vi "SLSC Convert Items - Variant to String.vi"(0 "dataType":string, 1 "format string":string="%#_12g", 5 "value":variant, 7 "min":variant, 9 "max":variant, 12 "string enums":T2(array[cluster])) -> (4 "Output data type":string, 6 "string offline data value":string, 8 "string min":string, 10 "string max":string, 14 "data_range":string)   [LabVIEW 2017, in "SLSC Tree Control.lvlib"]
doc: "Converts all of the item elements from variant into strings."
uses:
  SLSC Tree Control.lvlib
  Ctrl/EnumValue.ctl
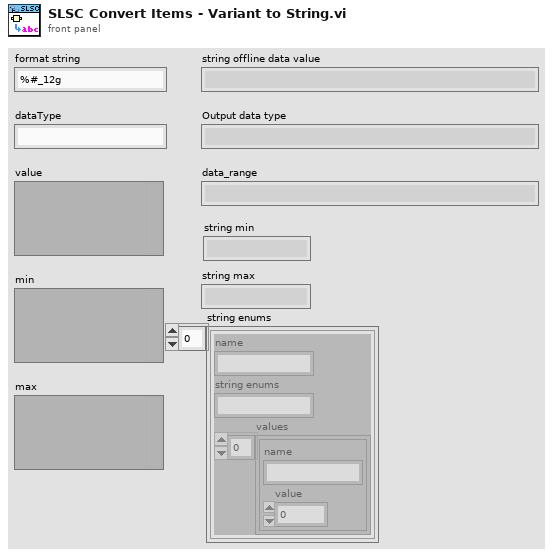
[diagram p1: front panel]
types:
  T1 = typedef "EnumValue.ctl" = cluster{"name":string, "value":i32}
  T2 = cluster{"name":string, "string enums":string, "values":T1[]}[]
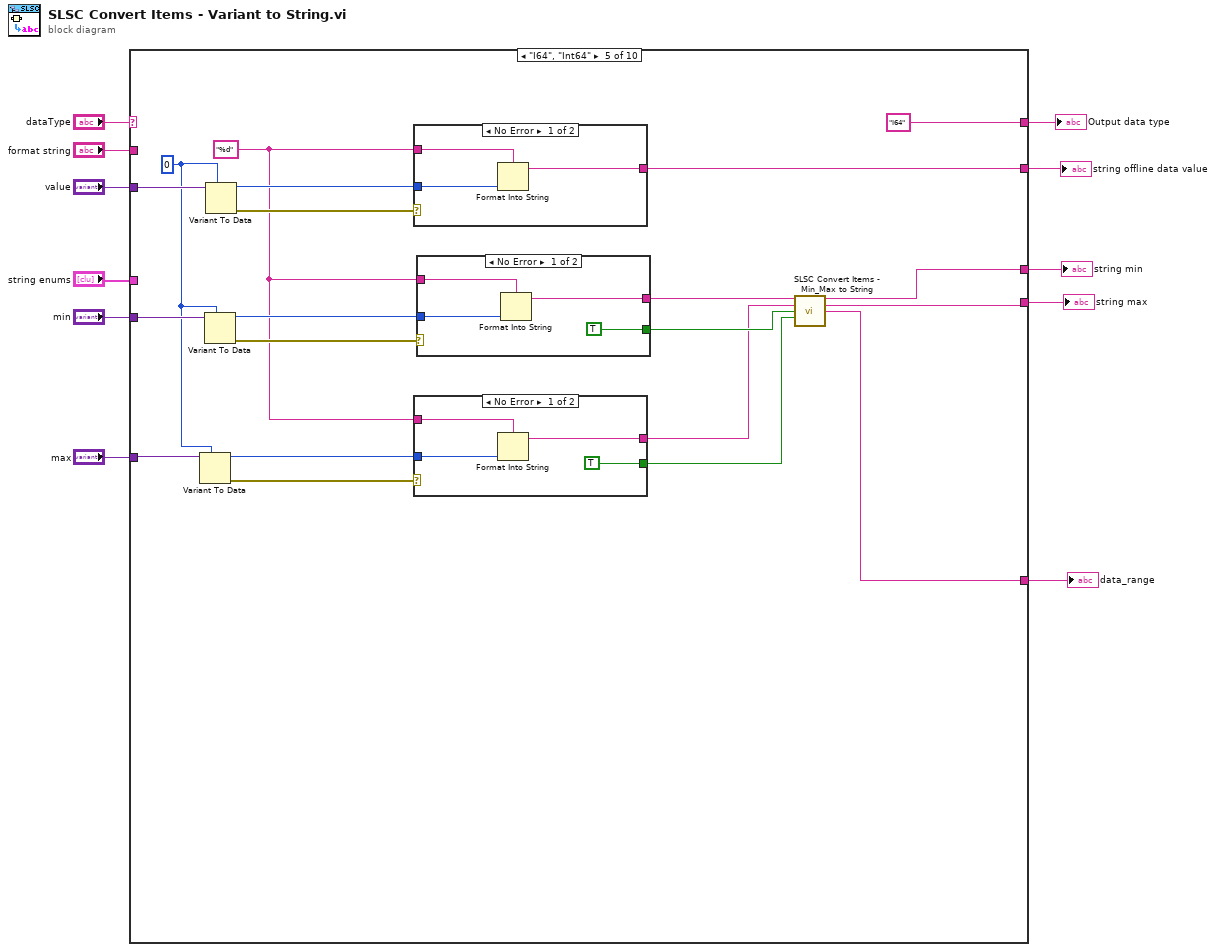
[diagram p0: block diagram]
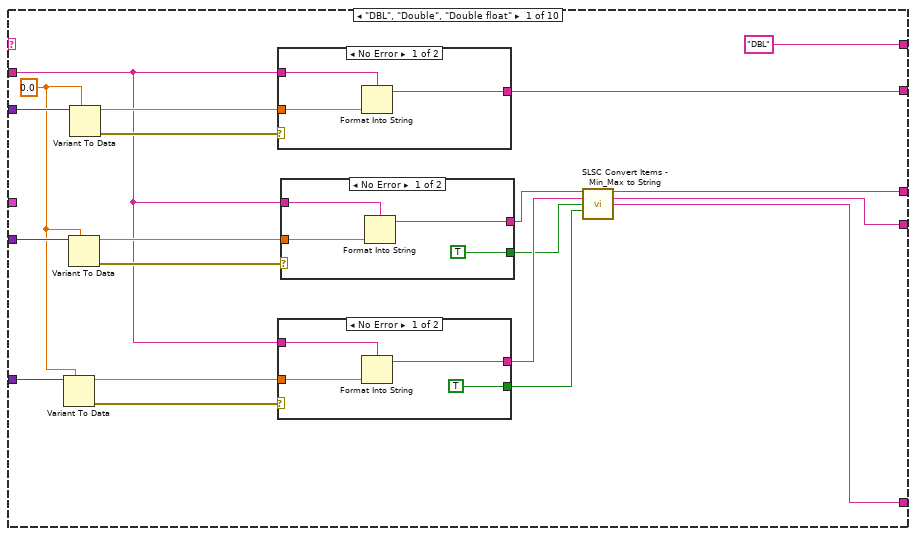
[diagram p2: hidden frame]
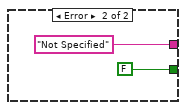
[diagram p3: hidden frame]
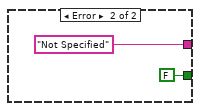
[diagram p4: hidden frame]
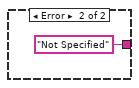
[diagram p5: hidden frame]
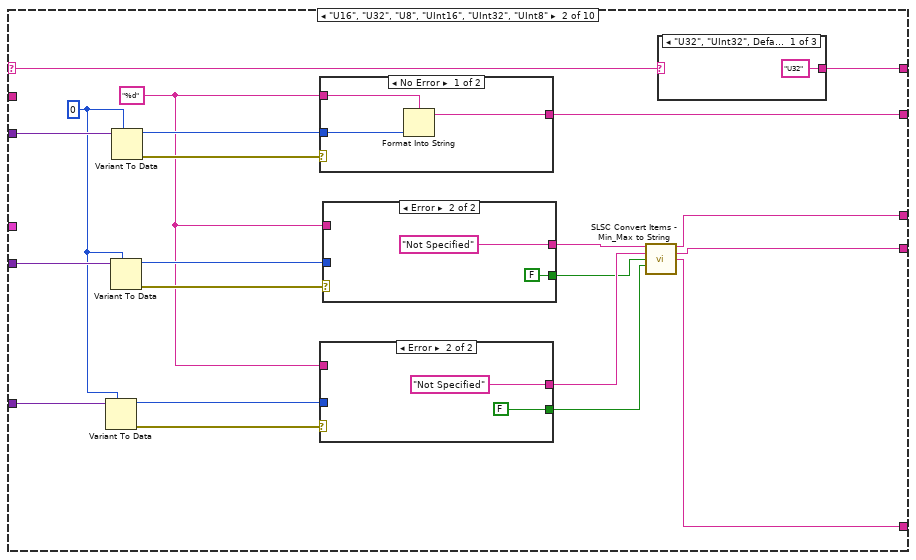
[diagram p6: hidden frame]
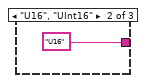
[diagram p7: hidden frame]
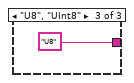
[diagram p8: hidden frame]
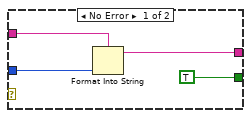
[diagram p9: hidden frame]
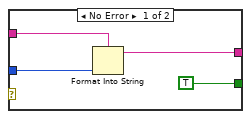
[diagram p10: hidden frame]
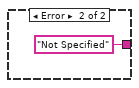
[diagram p11: hidden frame]
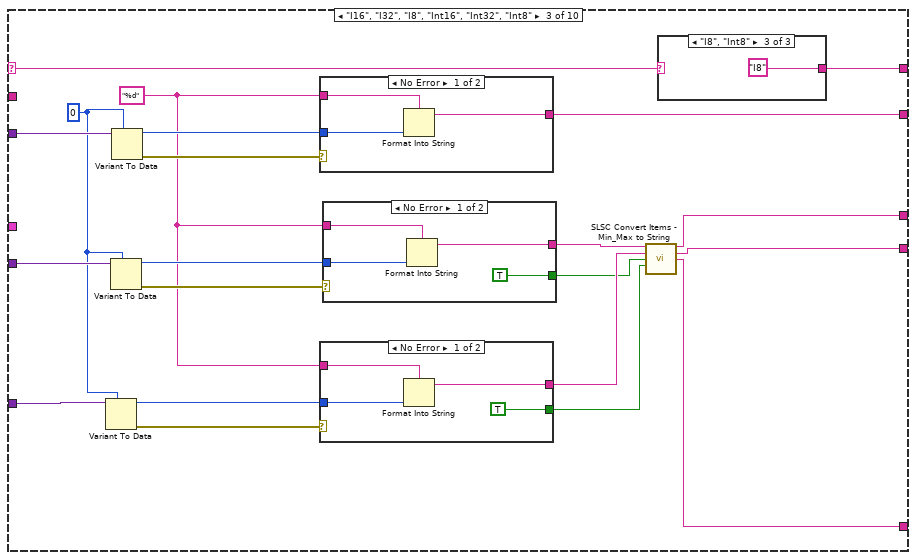
[diagram p12: hidden frame]
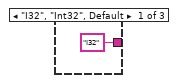
[diagram p13: hidden frame]
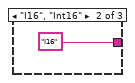
[diagram p14: hidden frame]
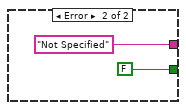
[diagram p15: hidden frame]
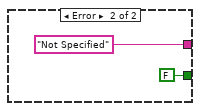
[diagram p16: hidden frame]
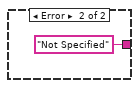
[diagram p17: hidden frame]
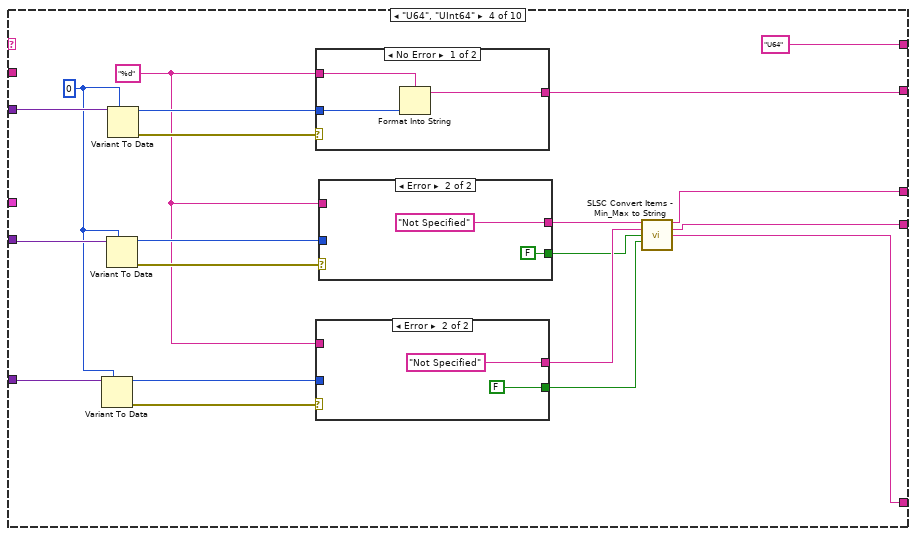
[diagram p18: hidden frame]
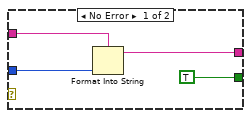
[diagram p19: hidden frame]
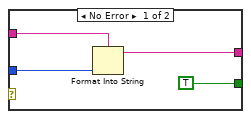
[diagram p20: hidden frame]
diagram:
  n1 = case shown="\"I64\", \"Int64\"" "dataType" {
    selector: "dataType" -> [_ w51 w91 _ _ _ w242 w248 w321 w403]
    tunnel: "value" -> [w31 w58 w98 w141 w174 w216 w241 w249 w322 w406]
    tunnel: [w23 w55 w95 w138 w167 w217 w240 w244 w317 w404] -> w4
    tunnel: ["DBL" w50 w90 "U64" "I64" "Bool" w242 w248 w321 w403] -> w9
    tunnel: "min" -> [w29 w57 w97 w140 w173 w212 _ w246 w319 w401]
    tunnel: "max" -> [w28 w56 w96 w139 w172 w210 _ w245 w318 w399]
    tunnel: [w26 w54 w94 w133 w182 w205 _ _ _ _] -> w6
    tunnel: [w25 w53 w93 w132 w181 w204 _ _ _ _] -> w5
    tunnel: "format string" -> [w12 _ _ _ _ _ _ _ _ _]
    tunnel: "string enums" -> [_ _ _ _ _ _ _ w247 w320 w405]
    tunnel: [w27 w52 w92 w131 w183 w203 _ w243 w316 w396] -> w11
    frame "DBL", "Double", "Double float" {
      w13 = 0.0
      n2 = Variant To Data(type=w13, Variant=w28) -> (data=w18:dbl, error out=w19:errorcluster)  [unwired: 1 in]
      n3 = Variant To Data(type=w13, Variant=w29) -> (data=w20:dbl, error out=w21:errorcluster)  [unwired: 1 in]
      n4 = Variant To Data(type=w13, Variant=w31) -> (data=w30:dbl, error out=w22:errorcluster)  [unwired: 1 in]
      n5 = case shown="No Error" w22 {
        tunnel: w30 -> [w46 _]
        tunnel: w12 -> [w45 _]
        tunnel: [w44 "Not Specified"] -> w23
        frame No Error {
          n6 = Format Into String(format string=w45, w46) -> (resulting string=w44:string)  [unwired: 2 in, 1 out]
        }
        frame Error {
        }
      }
      n7 = case shown="No Error" w19 {
        tunnel: w18 -> [w35 _]
        tunnel: w12 -> [w34 _]
        tunnel: [w33 "Not Specified"] -> w16
        tunnel: [TRUE ("min?") FALSE ("min?")] -> w14
        frame No Error {
          n8 = Format Into String(format string=w34, w35) -> (resulting string=w33:string)  [unwired: 2 in, 1 out]
        }
        frame Error {
        }
      }
      n9 = case shown="No Error" w21 {
        tunnel: w20 -> [w41 _]
        tunnel: w12 -> [w40 _]
        tunnel: [w39 "Not Specified"] -> w17
        tunnel: [TRUE ("min?") FALSE ("min?")] -> w15
        frame No Error {
          n10 = Format Into String(format string=w40, w41) -> (resulting string=w39:string)  [unwired: 2 in, 1 out]
        }
        frame Error {
        }
      }
      n11 = call "SLSC Convert Items - Min_Max to String.vi"("minimum"=w17, "maximum"=w16, "min?"=w15, "max?"=w14) -> ("minimum out"=w26:string, "maximum out"=w25:string, "minmax string"=w27:string)  [unwired: 9 in]
    }
    frame "U16", "U32", "U8", "UInt16", "UInt32", "UInt8" {
      w48 = "%d" ("format string")
      w49 = u32 0
      n12 = Variant To Data(type=w49, Variant=w56) -> (data=w63:u32, error out=w64:errorcluster)  [unwired: 1 in]
      n13 = Variant To Data(type=w49, Variant=w57) -> (data=w65:u32, error out=w66:errorcluster)  [unwired: 1 in]
      n14 = Variant To Data(type=w49, Variant=w58) -> (data=w68:u32, error out=w67:errorcluster)  [unwired: 1 in]
      n15 = case shown="No Error" w67 {
        tunnel: w68 -> [w86 _]
        tunnel: w48 -> [w85 _]
        tunnel: [w84 "Not Specified"] -> w55
        frame No Error {
          n16 = Format Into String(format string=w85, w86) -> (resulting string=w84:string)  [unwired: 2 in, 1 out]
        }
        frame Error {
        }
      }
      n17 = case shown="Error" w64 {
        tunnel: w63 -> [w75 _]
        tunnel: w48 -> [w74 _]
        tunnel: [w73 "Not Specified"] -> w61
        tunnel: [TRUE ("min?") FALSE ("min?")] -> w59
        frame No Error {
          n18 = Format Into String(format string=w74, w75) -> (resulting string=w73:string)  [unwired: 2 in, 1 out]
        }
        frame Error {
        }
      }
      n19 = case shown="Error" w66 {
        tunnel: w65 -> [w81 _]
        tunnel: w48 -> [w80 _]
        tunnel: [w79 "Not Specified"] -> w62
        tunnel: [TRUE ("min?") FALSE ("min?")] -> w60
        frame No Error {
          n20 = Format Into String(format string=w80, w81) -> (resulting string=w79:string)  [unwired: 2 in, 1 out]
        }
        frame Error {
        }
      }
      n21 = call "SLSC Convert Items - Min_Max to String.vi"("minimum"=w62, "maximum"=w61, "min?"=w60, "max?"=w59) -> ("minimum out"=w54:string, "maximum out"=w53:string, "minmax string"=w52:string)  [unwired: 9 in]
      n22 = case shown="\"U32\", \"UInt32\", Default" w51 {
        tunnel: ["U32" "U16" "U8"] -> w50
        frame "U32", "UInt32", Default {
        }
        frame "U16", "UInt16" {
        }
        frame "U8", "UInt8" {
        }
      }
    }
    frame "I16", "I32", "I8", "Int16", "Int32", "Int8" {
      w88 = "%d" ("format string")
      w89 = 0
      n23 = Variant To Data(type=w89, Variant=w96) -> (data=w103:i32, error out=w104:errorcluster)  [unwired: 1 in]
      n24 = Variant To Data(type=w89, Variant=w97) -> (data=w105:i32, error out=w106:errorcluster)  [unwired: 1 in]
      n25 = Variant To Data(type=w89, Variant=w98) -> (data=w108:i32, error out=w107:errorcluster)  [unwired: 1 in]
      n26 = case shown="No Error" w107 {
        tunnel: w108 -> [w126 _]
        tunnel: w88 -> [w125 _]
        tunnel: [w124 "Not Specified"] -> w95
        frame No Error {
          n27 = Format Into String(format string=w125, w126) -> (resulting string=w124:string)  [unwired: 2 in, 1 out]
        }
        frame Error {
        }
      }
      n28 = case shown="No Error" w104 {
        tunnel: w103 -> [w115 _]
        tunnel: w88 -> [w114 _]
        tunnel: [w113 "Not Specified"] -> w101
        tunnel: [TRUE ("min?") FALSE ("min?")] -> w99
        frame No Error {
          n29 = Format Into String(format string=w114, w115) -> (resulting string=w113:string)  [unwired: 2 in, 1 out]
        }
        frame Error {
        }
      }
      n30 = case shown="No Error" w106 {
        tunnel: w105 -> [w121 _]
        tunnel: w88 -> [w120 _]
        tunnel: [w119 "Not Specified"] -> w102
        tunnel: [TRUE ("min?") FALSE ("min?")] -> w100
        frame No Error {
          n31 = Format Into String(format string=w120, w121) -> (resulting string=w119:string)  [unwired: 2 in, 1 out]
        }
        frame Error {
        }
      }
      n32 = call "SLSC Convert Items - Min_Max to String.vi"("minimum"=w102, "maximum"=w101, "min?"=w100, "max?"=w99) -> ("minimum out"=w94:string, "maximum out"=w93:string, "minmax string"=w92:string)  [unwired: 9 in]
      n33 = case shown="\"I8\", \"Int8\"" w91 {
        tunnel: ["I32" "I16" "I8"] -> w90
        frame "I32", "Int32", Default {
        }
        frame "I16", "Int16" {
        }
        frame "I8", "Int8" {
        }
      }
    }
    frame "U64", "UInt64" {
      w128 = "%d" ("format string")
      w129 = u64 0
      n34 = Variant To Data(type=w129, Variant=w139) -> (data=w142:u64, error out=w143:errorcluster)  [unwired: 1 in]
      n35 = Variant To Data(type=w129, Variant=w140) -> (data=w144:u64, error out=w145:errorcluster)  [unwired: 1 in]
      n36 = Variant To Data(type=w129, Variant=w141) -> (data=w147:u64, error out=w146:errorcluster)  [unwired: 1 in]
      n37 = case shown="No Error" w146 {
        tunnel: w147 -> [w162 _]
        tunnel: w128 -> [w161 _]
        tunnel: [w160 "Not Specified"] -> w138
        frame No Error {
          n38 = Format Into String(format string=w161, w162) -> (resulting string=w160:string)  [unwired: 2 in, 1 out]
        }
        frame Error {
        }
      }
      n39 = case shown="Error" w143 {
        tunnel: w142 -> [w151 _]
        tunnel: w128 -> [w150 _]
        tunnel: [w149 "Not Specified"] -> w136
        tunnel: [TRUE ("min?") FALSE ("min?")] -> w134
        frame No Error {
          n40 = Format Into String(format string=w150, w151) -> (resulting string=w149:string)  [unwired: 2 in, 1 out]
        }
        frame Error {
        }
      }
      n41 = case shown="Error" w145 {
        tunnel: w144 -> [w157 _]
        tunnel: w128 -> [w156 _]
        tunnel: [w155 "Not Specified"] -> w137
        tunnel: [TRUE ("min?") FALSE ("min?")] -> w135
        frame No Error {
          n42 = Format Into String(format string=w156, w157) -> (resulting string=w155:string)  [unwired: 2 in, 1 out]
        }
        frame Error {
        }
      }
      n43 = call "SLSC Convert Items - Min_Max to String.vi"("minimum"=w137, "maximum"=w136, "min?"=w135, "max?"=w134) -> ("minimum out"=w133:string, "maximum out"=w132:string, "minmax string"=w131:string)  [unwired: 9 in]
    }
    frame "I64", "Int64" {
      w164 = "%d" ("format string")
      w165 = i64 0
      n44 = Variant To Data(type=w165, Variant=w172) -> (data=w175:i64, error out=w176:errorcluster)  [unwired: 1 in]
      n45 = Variant To Data(type=w165, Variant=w173) -> (data=w177:i64, error out=w178:errorcluster)  [unwired: 1 in]
      n46 = Variant To Data(type=w165, Variant=w174) -> (data=w180:i64, error out=w179:errorcluster)  [unwired: 1 in]
      n47 = case shown="No Error" w179 {
        tunnel: w180 -> [w198 _]
        tunnel: w164 -> [w197 _]
        tunnel: [w196 "Not Specified"] -> w167
        frame No Error {
          n48 = Format Into String(format string=w197, w198) -> (resulting string=w196:string)  [unwired: 2 in, 1 out]
        }
        frame Error {
        }
      }
      n49 = case shown="No Error" w176 {
        tunnel: w175 -> [w187 _]
        tunnel: w164 -> [w186 _]
        tunnel: [w185 "Not Specified"] -> w169
        tunnel: [TRUE ("min?") FALSE ("min?")] -> w168
        frame No Error {
          n50 = Format Into String(format string=w186, w187) -> (resulting string=w185:string)  [unwired: 2 in, 1 out]
        }
        frame Error {
        }
      }
      n51 = case shown="No Error" w178 {
        tunnel: w177 -> [w193 _]
        tunnel: w164 -> [w192 _]
        tunnel: [w191 "Not Specified"] -> w171
        tunnel: [TRUE ("min?") FALSE ("min?")] -> w170
        frame No Error {
          n52 = Format Into String(format string=w192, w193) -> (resulting string=w191:string)  [unwired: 2 in, 1 out]
        }
        frame Error {
        }
      }
      n53 = call "SLSC Convert Items - Min_Max to String.vi"("minimum"=w171, "maximum"=w169, "min?"=w170, "max?"=w168) -> ("minimum out"=w182:string, "maximum out"=w181:string, "minmax string"=w183:string)  [unwired: 9 in]
    }
    frame "Bool", "Boolean" {
      n54 = Equal?(x=w216, y=variant) -> (x = y?=w214:bool)
      n55 = Equal?(x=w210, y=variant) -> (x = y?=w207:bool)
      n56 = Equal?(x=w212, y=variant) -> (x = y?=w206:bool)
      n57 = Not(x=w207) -> (.not. x?=w200:bool)
      n58 = Not(x=w206) -> (.not. x?=w201:bool)
      n59 = case shown="True" w214 {
        tunnel: ["Not Specified" w236] -> w217
        tunnel: w216 -> [_ w233]
        frame True {
        }
        frame False {
          n60 = Variant To Data(type=FALSE, Variant=w233) -> (data=w234:bool)  [unwired: 1 in, 1 out]
          n61 = Select(t="True" ("data string"), s=w234, f="False" ("data string")) -> (s? t:f=w236:string)
        }
      }
      n62 = case shown="False" w207 {
        tunnel: ["Not Specified" w222] -> w208
        tunnel: w210 -> [_ w219]
        frame True {
        }
        frame False {
          n63 = Variant To Data(type=FALSE, Variant=w219) -> (data=w220:bool)  [unwired: 1 in, 1 out]
          n64 = Select(t="True" ("data string"), s=w220, f="False" ("data string")) -> (s? t:f=w222:string)
        }
      }
      n65 = case shown="False" w206 {
        tunnel: ["Not Specified" w229] -> w209
        tunnel: w212 -> [_ w226]
        frame True {
        }
        frame False {
          n66 = Variant To Data(type=FALSE, Variant=w226) -> (data=w227:bool)  [unwired: 1 in, 1 out]
          n67 = Select(t="True" ("data string"), s=w227, f="False" ("data string")) -> (s? t:f=w229:string)
        }
      }
      n68 = call "SLSC Convert Items - Min_Max to String.vi"("minimum"=w209, "maximum"=w208, "min?"=w201, "max?"=w200) -> ("minimum out"=w205:string, "maximum out"=w204:string, "minmax string"=w203:string)  [unwired: 9 in]
    }
    frame "String" {
      n69 = Variant To Data(type="" ("data string"), Variant=w241) -> (data=w240:string)  [unwired: 1 in, 1 out]
    }
    frame "NI.LEDState" {
      n70 = for {
        tunnel: w247 -> [w315] mode=indexing
        tunnel: w248 -> [w313]
        tunnel: [w310] -> w254 if=w312
        tunnel: [w312] -> _
        tunnel: [w311] -> w253
        stop <- w312 stop-if-true
        n71 = Unbundle By Name(w315) -> ("name"=w314:string, "values"=w311:T1[], "string enums"=w310:string)
        n72 = Equal?(x=w313, y=w314) -> (x = y?=w312:bool)
      }
      n73 = Variant To Data(type=0, Variant=w245) -> (data=w258:i32, error out=w260:errorcluster)  [unwired: 1 in]
      n74 = Variant To Data(type=0, Variant=w246) -> (data=w259:i32, error out=w261:errorcluster)  [unwired: 1 in]
      n75 = Unbundle By Name(w261) -> ("status"=w257:bool)
      n76 = Unbundle By Name(w260) -> ("status"=w256:bool)
      n77 = Variant To Data(type=0, Variant=w249) -> (data=w263:i32, error out=w262:errorcluster)  [unwired: 1 in]
      n78 = Or(x=w257, y=w256) -> (x .or. y?=w255:bool)
      n79 = case shown="True" w255 {
        tunnel: w257 -> [_ w277]
        tunnel: w253 -> [_ w276]
        tunnel: [w264 w274] -> w243
        tunnel: w259 -> [_ w272]
        tunnel: w256 -> [_ w267]
        tunnel: w258 -> [_ w266]
        tunnel: w254 -> [w264 _]
        frame False {
        }
        frame True {
          n80 = Not(x=w277) -> (.not. x?=w273:bool)
          n81 = Not(x=w267) -> (.not. x?=w269:bool)
          n82 = Select(t=w272, s=w273, f=-2147483648) -> (s? t:f=w270:i32)
          n83 = Select(t=w266, s=w269, f=2147483647) -> (s? t:f=w265:i32)
          n84 = for {
            tunnel: w276 -> [w285] mode=indexing
            tunnel: w270 -> [w283]
            tunnel: w265 -> [w284]
            shift-right: [w278] -> w274
            shift-left: "" -> [w279]
            n85 = Unbundle By Name(w285) -> ("name"=w280:string, "value"=w281:i32)
            n86 = In Range and Coerce(upper limit=w284, x=w281, lower limit=w283) -> (In Range?=w282:bool)  [unwired: 1 out]
            n87 = case shown="True" w282 {
              tunnel: w281 -> [_ w291]
              tunnel: w280 -> [_ w287]
              tunnel: [w286 w289] -> w278
              tunnel: w279 -> [w286 w288]
              frame False {
              }
              frame True {
                n88 = Format Into String(format string="%d", w291) -> (resulting string=w294:string)  [unwired: 2 in, 1 out]
                n89 = Concatenate Strings(w288, "[" ("string"), w294, "]" ("string"), w287, ";" ("string")) -> (w289:string)
              }
            }
          }
        }
      }
      n90 = case shown="No Error" w262 {
        tunnel: w263 -> [w297 _]
        tunnel: [w299 ""] -> w244
        tunnel: w253 -> [w298 _]
        frame No Error {
          n91 = for {
            tunnel: w298 -> [w308] mode=indexing
            tunnel: w297 -> [w306]
            tunnel: [w305] -> w296 if=w304
            stop <- w304 stop-if-true
            n92 = Unbundle By Name(w308) -> ("value"=w307:i32, "name"=w305:string)
            n93 = Equal?(x=w306, y=w307) -> (x = y?=w304:bool)
          }
          n94 = Format Into String(format string="%d", w297) -> (resulting string=w300:string)  [unwired: 2 in, 1 out]
          n95 = Concatenate Strings("[" ("string"), w300, "]" ("string"), w296) -> (w299:string)
        }
        frame Error {
        }
      }
    }
    frame "NI.EventDelay" {
      n96 = for {
        tunnel: w320 -> [w388] mode=indexing
        tunnel: w321 -> [w386]
        tunnel: [w383] -> w327 if=w385
        tunnel: [w385] -> _
        tunnel: [w384] -> w326
        stop <- w385 stop-if-true
        n97 = Unbundle By Name(w388) -> ("name"=w387:string, "values"=w384:T1[], "string enums"=w383:string)
        n98 = Equal?(x=w386, y=w387) -> (x = y?=w385:bool)
      }
      n99 = Variant To Data(type=0, Variant=w318) -> (data=w331:i32, error out=w333:errorcluster)  [unwired: 1 in]
      n100 = Variant To Data(type=0, Variant=w319) -> (data=w332:i32, error out=w334:errorcluster)  [unwired: 1 in]
      n101 = Unbundle By Name(w334) -> ("status"=w330:bool)
      n102 = Unbundle By Name(w333) -> ("status"=w329:bool)
      n103 = Variant To Data(type=0, Variant=w322) -> (data=w336:i32, error out=w335:errorcluster)  [unwired: 1 in]
      n104 = Or(x=w330, y=w329) -> (x .or. y?=w328:bool)
      n105 = case shown="True" w328 {
        tunnel: w330 -> [_ w350]
        tunnel: w326 -> [_ w349]
        tunnel: [w337 w347] -> w316
        tunnel: w332 -> [_ w345]
        tunnel: w329 -> [_ w340]
        tunnel: w331 -> [_ w339]
        tunnel: w327 -> [w337 _]
        frame False {
        }
        frame True {
          n106 = Not(x=w350) -> (.not. x?=w346:bool)
          n107 = Not(x=w340) -> (.not. x?=w342:bool)
          n108 = Select(t=w345, s=w346, f=-2147483648) -> (s? t:f=w343:i32)
          n109 = Select(t=w339, s=w342, f=2147483647) -> (s? t:f=w338:i32)
          n110 = for {
            tunnel: w349 -> [w358] mode=indexing
            tunnel: w343 -> [w356]
            tunnel: w338 -> [w357]
            shift-right: [w351] -> w347
            shift-left: "" -> [w352]
            n111 = Unbundle By Name(w358) -> ("name"=w353:string, "value"=w354:i32)
            n112 = In Range and Coerce(upper limit=w357, x=w354, lower limit=w356) -> (In Range?=w355:bool)  [unwired: 1 out]
            n113 = case shown="True" w355 {
              tunnel: w354 -> [_ w364]
              tunnel: w353 -> [_ w360]
              tunnel: [w359 w362] -> w351
              tunnel: w352 -> [w359 w361]
              frame False {
              }
              frame True {
                n114 = Format Into String(format string="%d", w364) -> (resulting string=w367:string)  [unwired: 2 in, 1 out]
                n115 = Concatenate Strings(w361, "[" ("string"), w367, "]" ("string"), w360, ";" ("string")) -> (w362:string)
              }
            }
          }
        }
      }
      n116 = case shown="No Error" w335 {
        tunnel: w336 -> [w370 _]
        tunnel: [w372 ""] -> w317
        tunnel: w326 -> [w371 _]
        frame No Error {
          n117 = for {
            tunnel: w371 -> [w381] mode=indexing
            tunnel: w370 -> [w379]
            tunnel: [w378] -> w369 if=w377
            stop <- w377 stop-if-true
            n118 = Unbundle By Name(w381) -> ("value"=w380:i32, "name"=w378:string)
            n119 = Equal?(x=w379, y=w380) -> (x = y?=w377:bool)
          }
          n120 = Format Into String(format string="%d", w370) -> (resulting string=w373:string)  [unwired: 2 in, 1 out]
          n121 = Concatenate Strings("[" ("string"), w373, "]" ("string"), w369) -> (w372:string)
        }
        frame Error {
        }
      }
    }
    frame Default {
      n122 = for {
        tunnel: w405 -> [w461] mode=indexing
        tunnel: w403 -> [w459]
        tunnel: [w456] -> w390 if=w458
        tunnel: [w458] -> _
        tunnel: [w457] -> w389
        stop <- w458 stop-if-true
        n123 = Unbundle By Name(w461) -> ("name"=w460:string, "values"=w457:T1[], "string enums"=w456:string)
        n124 = Equal?(x=w459, y=w460) -> (x = y?=w458:bool)
      }
      n125 = Variant To Data(type=0, Variant=w399) -> (data=w394:i32, error out=w397:errorcluster)  [unwired: 1 in]
      n126 = Variant To Data(type=0, Variant=w401) -> (data=w395:i32, error out=w398:errorcluster)  [unwired: 1 in]
      n127 = Unbundle By Name(w398) -> ("status"=w393:bool)
      n128 = Unbundle By Name(w397) -> ("status"=w392:bool)
      n129 = Variant To Data(type=0, Variant=w406) -> (data=w408:i32, error out=w407:errorcluster)  [unwired: 1 in]
      n130 = Or(x=w393, y=w392) -> (x .or. y?=w391:bool)
      n131 = case shown="True" w391 {
        tunnel: w393 -> [_ w423]
        tunnel: w389 -> [_ w422]
        tunnel: [w410 w420] -> w396
        tunnel: w395 -> [_ w418]
        tunnel: w392 -> [_ w413]
        tunnel: w394 -> [_ w412]
        tunnel: w390 -> [w410 _]
        frame False {
        }
        frame True {
          n132 = Not(x=w423) -> (.not. x?=w419:bool)
          n133 = Not(x=w413) -> (.not. x?=w415:bool)
          n134 = Select(t=w418, s=w419, f=-2147483648) -> (s? t:f=w416:i32)
          n135 = Select(t=w412, s=w415, f=2147483647) -> (s? t:f=w411:i32)
          n136 = for {
            tunnel: w422 -> [w431] mode=indexing
            tunnel: w416 -> [w429]
            tunnel: w411 -> [w430]
            shift-right: [w424] -> w420
            shift-left: "" -> [w425]
            n137 = Unbundle By Name(w431) -> ("name"=w426:string, "value"=w427:i32)
            n138 = In Range and Coerce(upper limit=w430, x=w427, lower limit=w429) -> (In Range?=w428:bool)  [unwired: 1 out]
            n139 = case shown="True" w428 {
              tunnel: w427 -> [_ w437]
              tunnel: w426 -> [_ w433]
              tunnel: [w432 w435] -> w424
              tunnel: w425 -> [w432 w434]
              frame False {
              }
              frame True {
                n140 = Format Into String(format string="%d", w437) -> (resulting string=w440:string)  [unwired: 2 in, 1 out]
                n141 = Concatenate Strings(w434, "[" ("string"), w440, "]" ("string"), w433, ";" ("string")) -> (w435:string)
              }
            }
          }
        }
      }
      n142 = case shown="No Error" w407 {
        tunnel: w408 -> [w443 _]
        tunnel: [w445 ""] -> w404
        tunnel: w389 -> [w444 _]
        frame No Error {
          n143 = for {
            tunnel: w444 -> [w454] mode=indexing
            tunnel: w443 -> [w452]
            tunnel: [w451] -> w442 if=w450
            stop <- w450 stop-if-true
            n144 = Unbundle By Name(w454) -> ("value"=w453:i32, "name"=w451:string)
            n145 = Equal?(x=w452, y=w453) -> (x = y?=w450:bool)
          }
          n146 = Format Into String(format string="%d", w443) -> (resulting string=w446:string)  [unwired: 2 in, 1 out]
          n147 = Concatenate Strings("[" ("string"), w446, "]" ("string"), w442) -> (w445:string)
        }
        frame Error {
        }
      }
    }
  }
  "data_range" <- w11
  "Output data type" <- w9
  "string offline data value" <- w4
  "string min" <- w6
  "string max" <- w5
